vi "DecodeGasData SubVI.vi"(4 "FlowUnit":u8, 5 "Re fPressureUnit":u8, 6 "RefTempUnit":u8, 7 "DensityUnitCode":u8) -> (0 "Flow Unit Comment":string, 1 "Ref Pressure Unit Comment":string, 2 "Temperature Unit Comment":string, 3 "Density Unit Comment":string)   [LabVIEW 2019]
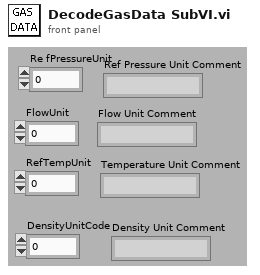
[diagram p1: front panel]
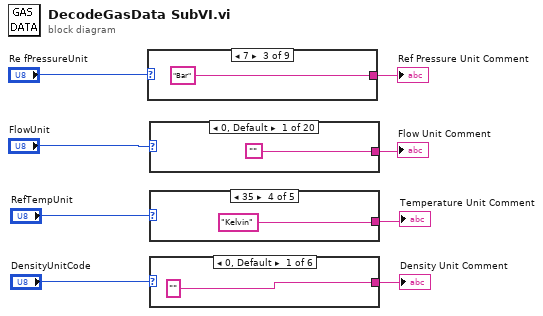
[diagram p0: block diagram]
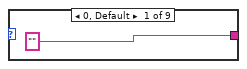
[diagram p2: hidden frame]
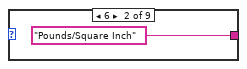
[diagram p3: hidden frame]
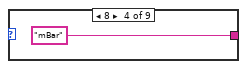
[diagram p4: hidden frame]
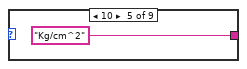
[diagram p5: hidden frame]
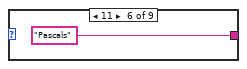
[diagram p6: hidden frame]
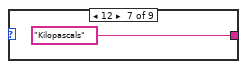
[diagram p7: hidden frame]
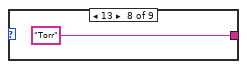
[diagram p8: hidden frame]
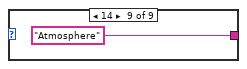
[diagram p9: hidden frame]
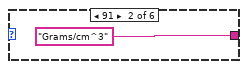
[diagram p10: hidden frame]
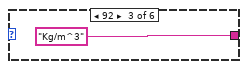
[diagram p11: hidden frame]
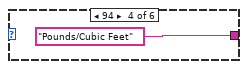
[diagram p12: hidden frame]
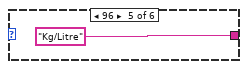
[diagram p13: hidden frame]
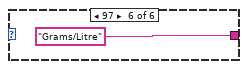
[diagram p14: hidden frame]
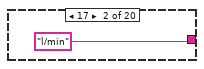
[diagram p15: hidden frame]
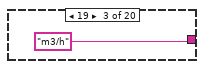
[diagram p16: hidden frame]
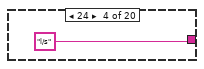
[diagram p17: hidden frame]
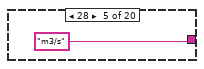
[diagram p18: hidden frame]
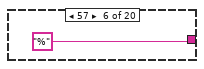
[diagram p19: hidden frame]
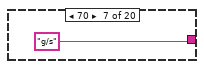
[diagram p20: hidden frame]
diagram:
  n1 = case shown="7" "Re fPressureUnit" {
    tunnel: ["" "Pounds/Square Inch" "Bar" "mBar" "Kg/cm^2" "Pascals" "Kilopascals" "Torr" "Atmosphere"] -> w2
    frame 0, Default {
    }
    frame 6 {
    }
    frame 7 {
    }
    frame 8 {
    }
    frame 10 {
    }
    frame 11 {
    }
    frame 12 {
    }
    frame 13 {
    }
    frame 14 {
    }
  }
  "Ref Pressure Unit Comment" <- w2
  n2 = case shown="0, Default" "FlowUnit" {
    tunnel: ["" "l/min" "m3/h" "l/s" "m3/s" "%" "g/s" "g/min" "g/h" "kg/s" "kg/min" "kg/h" "lbs/s" "lbs/min" "lbs/h" "m3/min" "l/h" "ml/s" "ml/min" "ml/h"] -> w7
    frame 0, Default {
    }
    frame 17 {
    }
    frame 19 {
    }
    frame 24 {
    }
    frame 28 {
    }
    frame 57 {
    }
    frame 70 {
    }
    frame 71 {
    }
    frame 72 {
    }
    frame 73 {
    }
    frame 74 {
    }
    frame 75 {
    }
    frame 80 {
    }
    frame 81 {
    }
    frame 82 {
    }
    frame 131 {
    }
    frame 138 {
    }
    frame 170 {
    }
    frame 171 {
    }
    frame 172 {
    }
  }
  "Flow Unit Comment" <- w7
  n3 = case shown="35" "RefTempUnit" {
    tunnel: ["Normal 273.15 Kelvin & 1013.33 mBar" "degC" "degF" "Kelvin" "As Defined at Calibration"] -> w8
    frame 0, Default {
    }
    frame 32 {
    }
    frame 33 {
    }
    frame 35 {
    }
    frame 2 {
    }
  }
  "Temperature Unit Comment" <- w8
  n4 = case shown="0, Default" "DensityUnitCode" {
    tunnel: ["" "Grams/cm^3" "Kg/m^3" "Pounds/Cubic Feet" "Kg/Litre" "Grams/Litre"] -> w4
    frame 0, Default {
    }
    frame 91 {
    }
    frame 92 {
    }
    frame 94 {
    }
    frame 96 {
    }
    frame 97 {
    }
  }
  "Density Unit Comment" <- w4
